vi "Generate File Name.vi"(11 "properties":cluster{"Key":string, "Value":string}[](array[cluster])) -> (3 "Array":cluster{"Key":string, "Value":string}[](array[cluster]))   [LabVIEW 2016]
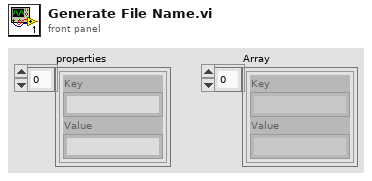
[diagram p1: front panel]
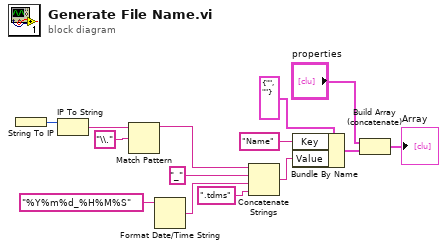
[diagram p0: block diagram]
diagram:
  n1 = String To IP() -> (0:w10:u32)  [unwired: 1 in]
  n2 = IP To String(2:w10) -> (0:w8:string)  [unwired: 1 in]
  n3 = Match Pattern(string=w8, regular expression="\\.") -> (before substring=w6:string)  [unwired: 1 in, 3 out]
  n4 = Format Date/Time String(time format string (%c)="%Y%m%d_%H%M%S") -> (date/time string=w9:string)  [unwired: 2 in]
  n5 = Concatenate Strings(w6, "_" ("string"), w9, ".tdms" ("string")) -> (w14:string)
  n6 = Bundle By Name(cluster=cluster{"Key":string, "Value":string} {"Key"="", "Value"=""} ("Property"), "Key"="Name" ("element"), "Value"=w14) -> (w2:cluster{"Key":string, "Value":string})
  n7 = Build Array (concatenate)("properties", w2) -> (→"Array":cluster{"Key":string, "Value":string}[])
